vi "Controller.vi"(0 "ControllerGains":T1, 1 "Current State":i32[](array[numeric]), 2 "MyID":u8, 3 "Pose":dbl[](array[numeric]), 4 "Feedback elements In":T2, 5 "CurrentWP":i32[](array[numeric]), 6 "Vref":dbl[](array[numeric]), 7 "Trajectory":dbl[][](array[numeric]), 14 "ActualTime":u32) -> (11 "Feedback elements Out":T2, 12 "v_real":dbl, 15 "Controls":u8[](array[numeric]))   [LabVIEW 2013]
uses:
  Global.vi
  <vilib>/imath/engines/lvmath2/RunTimeEngine/ErrorHandling/NIMS_Finalize Error.vi
  <vilib>/imath/engines/lvmath2/RunTimeEngine/IndexRead/NIMS V(S).vi
  <instcachedir>/0/NIMS V(S)_0488751826AF41519A22953C041130DC.lvgen/NIMS V(S)_0488751826AF41519A22953C041130DC_000.vi
  <vilib>/imathl/engines/lvmath/Functions/Error Handling/Create Error.vi
  <vilib>/imath/engines/lvmath2/RunTimeEngine/RunTimeType/NIMS_RunTimeType_From StrictType (excl LVString).vi
  <instcachedir>/0/NIMS_RunTimeType_From StrictType (excl LVString)_4DEE718D6EB74582AA20236969C084FC.lvgen/NIMS_RunTimeType_From StrictType (excl LVString)_4DEE718D6EB74582AA20236969C084FC_031.vi
  <vilib>/imath/engines/lvmath2/RunTimeEngine/Struct/NIMS_StructSetField.vi
  <vilib>/imath/engines/lvmath2/RunTimeEngine/NodeEndStatement/NIMS_NodeEndStatement_Output.vi
  <instcachedir>/0/NIMS_NodeEndStatement_Output_53EC0D466D134D7ABD903AC30B43404B.lvgen/NIMS_NodeEndStatement_Output_53EC0D466D134D7ABD903AC30B43404B_005.vi
  <instcachedir>/0/NIMS_NodeEndStatement_Output_53EC0D466D134D7ABD903AC30B43404B.lvgen/NIMS_NodeEndStatement_Output_53EC0D466D134D7ABD903AC30B43404B_013.vi
  <instcachedir>/0/NIMS_NodeEndStatement_Output_53EC0D466D134D7ABD903AC30B43404B.lvgen/NIMS_NodeEndStatement_Output_53EC0D466D134D7ABD903AC30B43404B_001.vi
  <instcachedir>/0/NIMS_NodeEndStatement_Output_53EC0D466D134D7ABD903AC30B43404B.lvgen/NIMS_NodeEndStatement_Output_53EC0D466D134D7ABD903AC30B43404B_009.vi
  <vilib>/imath/engines/lvmath2/RunTimeEngine/BuiltInFunctions/is_nan/NIMS_is_nan.vi
  <instcachedir>/0/NIMS_is_nan_BCCD798162CC49E3A8E57072444F6EB6.lvgen/NIMS_is_nan_BCCD798162CC49E3A8E57072444F6EB6_002.vi
  <instcachedir>/0/NIMS V(S)_0488751826AF41519A22953C041130DC.lvgen/NIMS V(S)_0488751826AF41519A22953C041130DC_002.vi
  <vilib>/imath/engines/lvmath/Functions/Error Handling/MergeErrorsWrapper.vi
  <vilib>/imath/engines/lvmath2/RunTimeEngine/Struct/NIMS_StructGetField.vi
  <vilib>/imath/engines/lvmath2/RunTimeEngine/RunTimeType/NIMS_RunTimeType_To Numeric.vi
  <instcachedir>/0/NIMS_RunTimeType_To Numeric_4795FB10E831402FABFA341B47E20681.lvgen/NIMS_RunTimeType_To Numeric_4795FB10E831402FABFA341B47E20681_008.vi
  <vilib>/imath/engines/lvmath2/RunTimeEngine/IndexRead/NIMS M(S,S).vi
  <instcachedir>/0/NIMS M(S,S)_AC51E74150A542F7991B9634C66F3096.lvgen/NIMS M(S,S)_AC51E74150A542F7991B9634C66F3096_000.vi
  <vilib>/imath/engines/lvmath2/RunTimeEngine/ErrorHandling/NIMS_Create Error From Enums.vi
  <vilib>/imath/engines/lvmath2/RunTimeEngine/BuiltInFunctions/atan2/NIMS_atan2.vi
  <instcachedir>/0/NIMS_atan2_A91AA4A7D42247EDBE8F76DB99AF04A4.lvgen/NIMS_atan2_A91AA4A7D42247EDBE8F76DB99AF04A4_000.vi
  <vilib>/imath/engines/lvmath2/RunTimeEngine/BuiltInFunctions/deg_to_rad/NIMS_deg_to_rad.vi
  <instcachedir>/0/NIMS_deg_to_rad_4A81D684CE8D4DD79924F5AB74D756E1.lvgen/NIMS_deg_to_rad_4A81D684CE8D4DD79924F5AB74D756E1_001.vi
  <vilib>/imath/engines/lvmath2/RunTimeEngine/BuiltInFunctions/rem/NIMS_rem_no checks.vi
  <instcachedir>/0/NIMS_rem_no checks_7935C26835844EFC868069820ED089DA.lvgen/NIMS_rem_no checks_7935C26835844EFC868069820ED089DA_000.vi
  <instcachedir>/0/NIMS_is_nan_BCCD798162CC49E3A8E57072444F6EB6.lvgen/NIMS_is_nan_BCCD798162CC49E3A8E57072444F6EB6_004.vi
  <vilib>/imath/engines/lvmath2/RunTimeEngine/IndexReplace/NIMS V(S)=S.vi
  <instcachedir>/0/NIMS V(S)=S_66A18068148B4981A312229A93EA5C06.lvgen/NIMS V(S)=S_66A18068148B4981A312229A93EA5C06_000.vi
  <vilib>/imath/engines/lvmath2/RunTimeEngine/BuiltInFunctions/round/NIMS_round(CDB-S).vi
  <vilib>/imath/engines/lvmath2/RunTimeEngine/BuiltInFunctions/rad_to_deg/NIMS_rad_to_deg.vi
  <instcachedir>/0/NIMS_rad_to_deg_A39AFCDDC8C049FCADAAB7FC30B9F5AA.lvgen/NIMS_rad_to_deg_A39AFCDDC8C049FCADAAB7FC30B9F5AA_001.vi
  <vilib>/imath/engines/lvmath2/RunTimeEngine/BuiltInFunctions/round/NIMS_round(DBL-S).vi
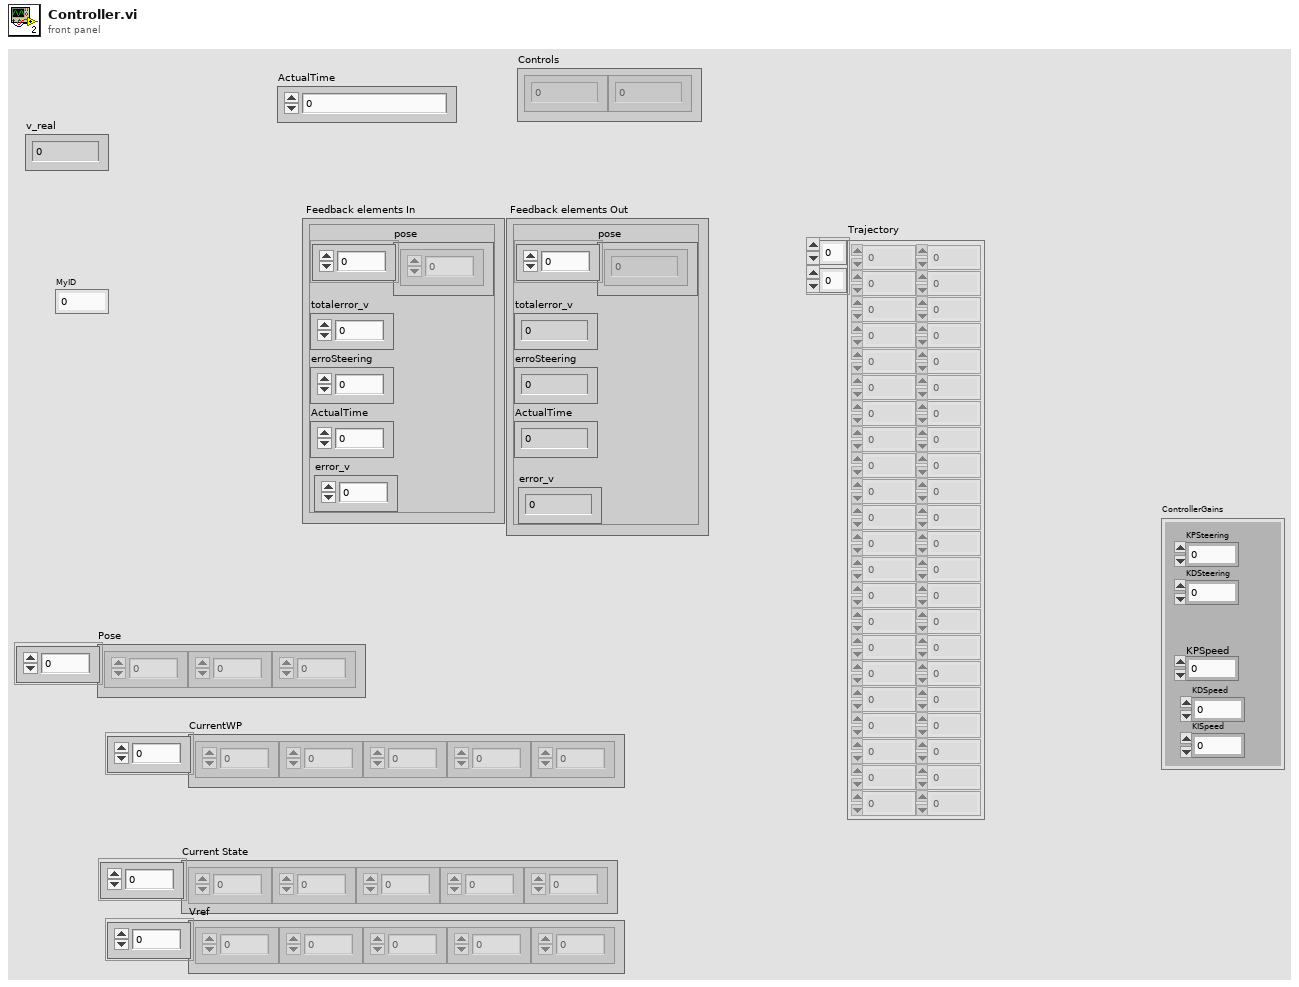
[diagram p1: front panel]
types:
  T1 = cluster{"KPSteering":dbl, "KDSteering":dbl, "KPSpeed":dbl, "KISpeed":dbl, "KDSpeed":dbl}
  T2 = cluster{"pose":dbl[], "totalerror_v":dbl, "erroSteering":dbl, "ActualTime":dbl, "error_v":dbl}
  T3 = cluster{"pose":dbl[], "totalerror_v":cdb, "erroSteering":dbl, "ActualTime":u32, "error_v":cdb}
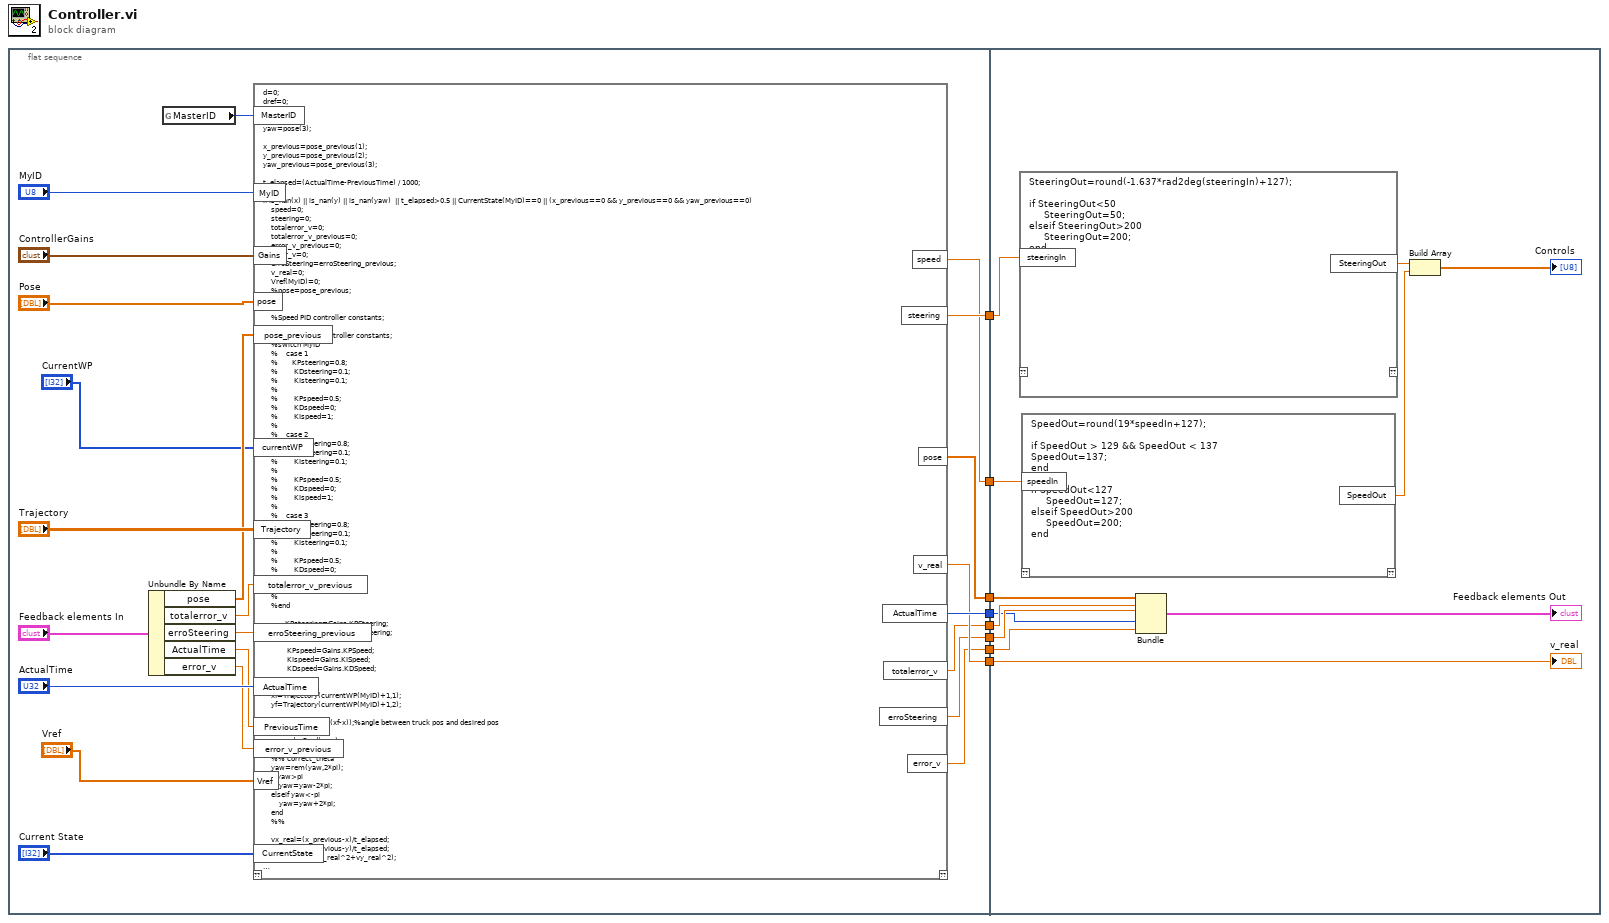
[diagram p0: block diagram]
diagram:
  n1 = flat-sequence {
    tunnel: [w15] -> w8
    tunnel: [w31] -> w7
    tunnel: [w30] -> w6
    tunnel: [w28] -> w5
    tunnel: [w26] -> w4
    tunnel: [w25] -> w3
    tunnel: [w22] -> w2
    tunnel: [w12] -> w1
    tunnel: w8 -> [w877]
    tunnel: w7 -> [w880]
    tunnel: w6 -> [w879]
    tunnel: w5 -> [w875]
    tunnel: w4 -> [w878]
    tunnel: w3 -> [w870]
    tunnel: w2 -> [w876]
    tunnel: w1 -> [w869]
    frame #0 {
      n2 = Unbundle By Name("Feedback elements In") -> ("pose"=w16:dbl[], "totalerror_v"=w21:dbl, "erroSteering"=w20:dbl, "ActualTime"=w19:dbl, "error_v"=w11:dbl)
      n3 = global read "Global.vi" "MasterID"() -> (w23:i32)
      n4 = mathscript code="d=0;\ndref=0;\nx=pose(1);\ny=pose(2);\nyaw=pose(3);\n\nx_previous=pose_previous(1);\ny_previous=pose_previous(2);\nyaw_previous=pose_previous(3);\n\nt_elapsed=(ActualTime-PreviousTime) / 1000;\n\nif is_nan(x) || is_nan(y) || is_nan(yaw)  || t_elapsed>0.5 || CurrentState(MyID)==0 || (x_previous==0 && y_previous==0 && yaw_previous==0)\n    speed=0;\n    steering=0;\n    totalerror_v=0;\n    totalerror_v_previous=0;\n    error_v_previous=0;\n    error_v=0;\n    erroSteering=erroSteering_previous;\n    v_real=0;\n    Vref(MyID)=0;\n    %pose=pose_previous;\nelse\n    \n    %Speed PID controller constants;\n    \n    %Steering PID controller constants;\n    %switch MyID\n    %    case 1\n    %       KPsteering=0.8;\n    %        KDsteering=0.1;\n    %        KIsteering=0.1;\n    %        \n    %        KPspeed=0.5;\n    %        KDspeed=0;\n    %        KIspeed=1;\n    %        \n    %    case 2\n    %        KPsteering=0.8;\n    %        KDsteering=0.1;\n    %        KIsteering=0.1;\n    %        \n    %        KPspeed=0.5;\n    %        KDspeed=0;\n    %        KIspeed=1;\n    %        \n    %    case 3\n    %        KPsteering=0.8;\n    %        KDsteering=0.1;\n    %        KIsteering=0.1;\n    %        \n    %        KPspeed=0.5;\n    %        KDspeed=0;\n    %        KIspeed=1;\n    %        \n    %        \n    %end\n\n           KPsteering=Gains.KPSteering;\n            KDsteering=Gains.KDSteering;\n            \n            KPspeed=Gains.KPSpeed;\n            KIspeed=Gains.KISpeed;\n            KDspeed=Gains.KDSpeed;\n    \n    \n    xf=Trajectory(currentWP(MyID)+1,1);\n    yf=Trajectory(currentWP(MyID)+1,2);\n    \n    phi=atan2((yf-y),(xf-x));%angle between truck pos and desired pos\n    \n    yaw=deg2rad(yaw);\n    \n    %% correct_theta\n    yaw=rem(yaw,2*pi);\n    if yaw>pi\n        yaw=yaw-2*pi;\n    elseif yaw<-pi\n        yaw=yaw+2*pi;\n    end\n    %% \n    \n    vx_real=(x_previous-x)/t_elapsed;\n    vy_real=(y_previous-y)/t_elapsed;\n    v_real=sqrt(vx_real^2+vy_real^2);\n    \n    if Vref(MyID)==0\n        totalerror_v_previous=0;\n        error_v_previous=0;\n        error_v=0;\n    end\n    \n    error_v=Vref(MyID)-v_real;\n    \n    totalerror_v=totalerror_v_previous+error_v*t_elapsed;\n    \n    if totalerror_v<0 || is_nan(totalerror_v)\n        totalerror_v=0;\n        error_v_previous=0;\n        error_v=0;\n    end\n    \n    erroSteering=phi-yaw;\n    \n    %% correct_theta\n    erroSteering=rem(erroSteering,2*pi);\n    if erroSteering>pi\n        erroSteering=erroSteering-2*pi;\n    elseif erroSteering<-pi\n        erroSteering=erroSteering+2*pi;\n    end\n    %%\n    \n    \n    speed=KPspeed*error_v + KIspeed*totalerror_v+KDspeed*(error_v-error_v_previous)/t_elapsed;\n    steering=KPsteering*erroSteering+KDsteering*(erroSteering-erroSteering_previous)/t_elapsed;\n    \n    %if erropos<0.5\n    %    currentWP=rem(currentWP+1, length(Trajectory));\n    %end\n    \nend"("totalerror_v_previous"=w21, "erroSteering_previous"=w20, "ActualTime"="ActualTime", "PreviousTime"=w19, "Trajectory"="Trajectory", "pose"="Pose", "pose_previous"=w16, "Vref"="Vref", "MyID"="MyID", "MasterID"=w23, "currentWP"="CurrentWP", "CurrentState"="Current State", "Gains"="ControllerGains", "error_v_previous"=w11) -> ("erroSteering"=w22:dbl, "speed"=w30:cdb, "steering"=w31:dbl, "ActualTime"=w28:u32, "pose"=w26:dbl[], "v_real"=w25:dbl, "totalerror_v"=w15:cdb, "error_v"=w12:cdb)  [unwired: 1 in, 1 out]
    }
    frame #1 {
      n5 = mathscript code="SteeringOut=round(-1.637*rad2deg(steeringIn)+127);\n\nif SteeringOut<50\n     SteeringOut=50;\nelseif SteeringOut>200\n     SteeringOut=200;\nend"("steeringIn"=w880) -> ("SteeringOut"=w873:dbl)  [unwired: 1 in, 1 out]
      n6 = mathscript code="SpeedOut=round(19*speedIn+127);\n\nif SpeedOut > 129 && SpeedOut < 137\nSpeedOut=137;\nend\n\nif SpeedOut<127\n     SpeedOut=127;\nelseif SpeedOut>200\n     SpeedOut=200;\nend"("speedIn"=w879) -> ("SpeedOut"=w872:cdb)  [unwired: 1 in, 1 out]
      n7 = Bundle("pose"=w878, "totalerror_v"=w877, "erroSteering"=w876, "ActualTime"=w875, "error_v"=w869) -> (→"Feedback elements Out":T3)  [unwired: 1 in]
      n8 = Build Array(w873, w872) -> (→"Controls":cdb[])
      "v_real" <- w870
    }
  }
